vi "Stack Tote.vi"(8 "error in":errorcluster, 9 "Auto Notifiers In":T1) -> (0 "error out(no error)":errorcluster, 1 "Auto Notifiers Out":T1)   [LabVIEW 2014]
doc: "This VI will wait on the TOTE limit switch to be hit signifying that that a tote is within our robot, after it has insured that a tote is within the robot it brings the elevator to the ground state."
uses:
  Auto Notifiers.ctl
  Main/Arms/Arm clapper state.ctl
  Main/Arms/Arm State.ctl
  Main/Elevator/Elevator States.ctl
  Utilities/Sensor Refname.ctl
  Utilities/Sensor Refname to String.vi
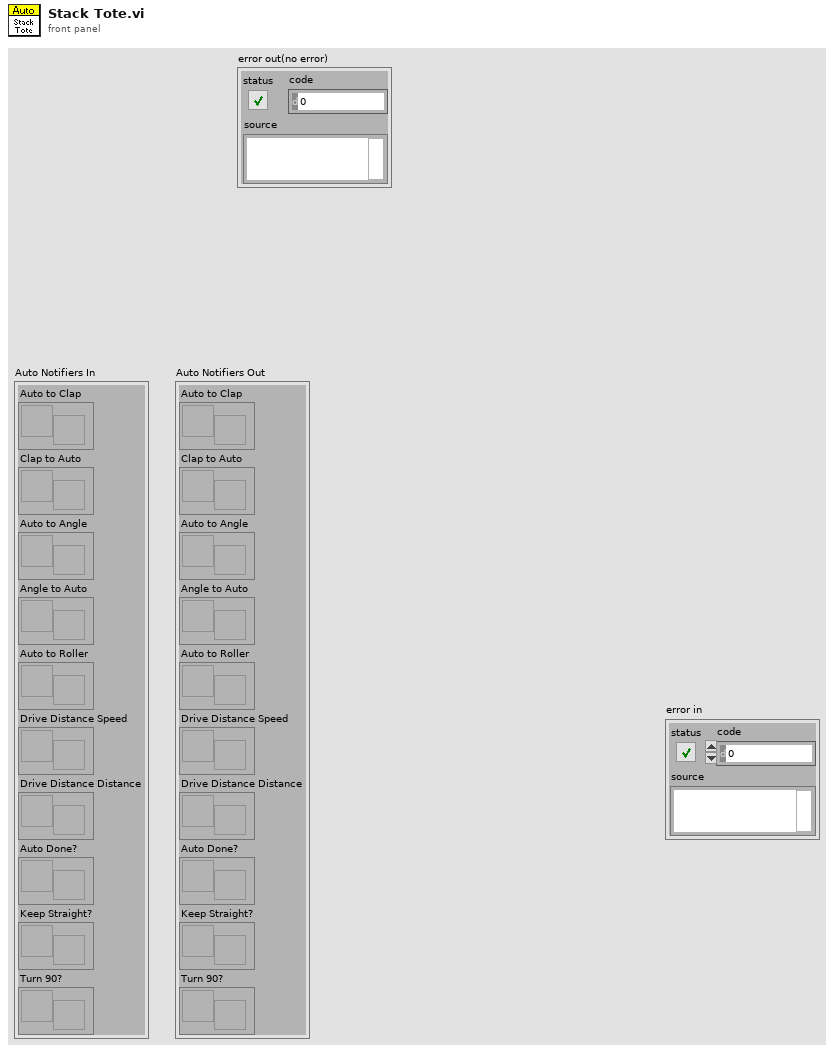
[diagram p1: front panel]
types:
  T1 = typedef "Auto Notifiers.ctl" = cluster{"Auto to Clap":refnum<notifier>, "Clap to Auto":refnum<notifier>, "Auto to Angle":refnum<notifier>, "Angle to Auto":refnum<notifier>, "Auto to Roller":refnum<notifier>, "Drive Distance Speed":refnum<notifier>, "Drive Distance Distance":refnum<notifier>, "Auto Done?":refnum<notifier>, "Keep Straight?":refnum<notifier>, "Turn 90?":refnum<notifier>}
  T2 = typedef "Elevator States.ctl" = enum16{"Ground", "Tote 1", "Tote 2", "Tote 3", "Tote 4", "Tote 5", "Tote 6"}
  T3 = typedef "Sensor Refname.ctl" = enum16{"Gyro", "Elevator Top LS", "Elevator Bottom LS", "Claw Outside LS", "Left Drive Encoder", "Right Drive Encoder", "Strafe Encoder", "Elevator Encoder", "Ultrasonic Forward", "Ultrasonic Back", "Arm Angle POT", "Arm Clapper POT", "Accelerometer", "Tote LS", "DIP 1", "DIP 2", "DIP 3", "DIP 4"}
  T4 = typedef "WPI_SwitchDevRef.ctl" = cluster{"DevStatus":errorcluster, "DIO Channel":T5, "Controller":T6, "CntIndex":T7, "Normally Closed":bool}
  T5 = typedef "FPGA_DIOChannel.ctl" = enum8{"DIO 0", "DIO 1", "DIO 2", "DIO 3", "DIO 4", "DIO 5", "DIO 6", "DIO 7", "DIO 8", "DIO 9", "DIO MXP 0", "DIO MXP 1", "DIO MXP 2", "DIO MXP 3", "DIO MXP 4", "DIO MXP 5", "DIO MXP 6", "DIO MXP 7", "DIO MXP 8", "DIO MXP 9", "DIO MXP 10", "DIO MXP 11", "DIO MXP 12", "DIO MXP 13", "DIO MXP 14", "DIO MXP 15", "Invalid"}
  T6 = typedef "FPGA_TypedefDigitalModule.ctl" = enum16{"Controller 1"}
  T7 = typedef "FPGA_CounterCtrSystemIndex.ctl" = enum8{"Ctr 0", "Ctr 1", "Ctr 2", "Ctr 3", "Ctr 4", "Ctr 5", "Ctr 6", "Ctr 7", "Invalid"}
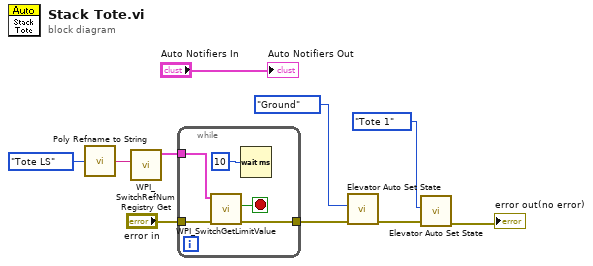
[diagram p0: block diagram]
diagram:
  n1 = call-poly "Poly Refname to String.vi"("Sensor Refnames"=Sensor_Refname."Tote LS") -> ("Refname"=w8:string)
  n2 = call <vilib>:"WPI_SwitchRefNum Registry Get.vi"("refnum name"=w8) -> ("SwitchDevRef"=w7:T4)  [unwired: 9 in, 1 out]
  n3 = while {
    tunnel: "error in" -> [w12]
    tunnel: [w13] -> w5
    tunnel: w7 -> [w14]
    stop <- w15 stop-if-true
    n4 = call <vilib>:"WPI_SwitchGetLimitValue.vi"("error in (no error)"=w12, "SwitchDevRef"=w14) -> ("error out"=w13:errorcluster, "Switch Pressed"=w15:bool)  [unwired: 7 in, 1 out]
    n5 = Wait (ms)(milliseconds to wait=u32 10) -> ()  [unwired: 1 out]
  }
  n6 = call "Elevator Auto Set State.vi"("error in (no error)"=w5, "New State"=Elevator_States."Ground" ("Elevator State")) -> ("error out"=w3:errorcluster)  [unwired: 9 in]
  n7 = call "Elevator Auto Set State.vi"("error in (no error)"=w3, "New State"=Elevator_States."Tote 1" ("Elevator State")) -> ("error out"=→"error out(no error)":errorcluster)  [unwired: 9 in]
  "Auto Notifiers Out" <- "Auto Notifiers In"
